vi "Rigol_DG4102.vi"(0 "VISA Refnum in":refnum<visa-resource-name>, 1 "Массив диода":dbl[](array[numeric]), 2 "Масиив детектора":dbl[](array[numeric]), 5 "Количество точек":i32, 7 "Частота (1000 Hz)":dbl=1000.0, 9 "Amplitude (5 Vpp)":dbl=5.0, 12 "Amplitude Unit (0: Vpp)":i32(ring) items=["Vpp", "Vrms", "dBm"], 13 "Amplitude Unit (0: Vpp) 2":i32(ring) items=["Vpp", "Vrms", "dBm"], 14 "Amplitude (5 Vpp) 2":dbl=5.0) -> (3 "VISA resource name out":refnum<visa-resource-name>, 4 "Выход на канал 1":string, 6 "Выход на канал 2":string)   [LabVIEW 2012]
uses:
  RIGOL DG4000 Series.lvlib
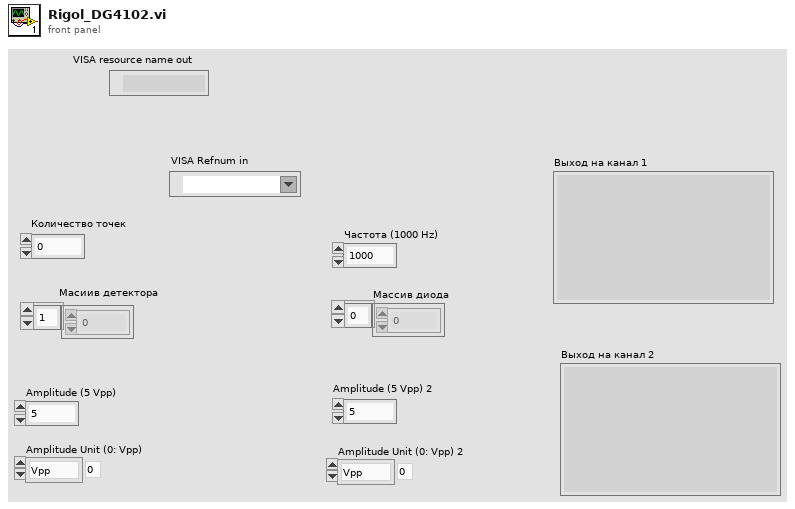
[diagram p1: front panel]
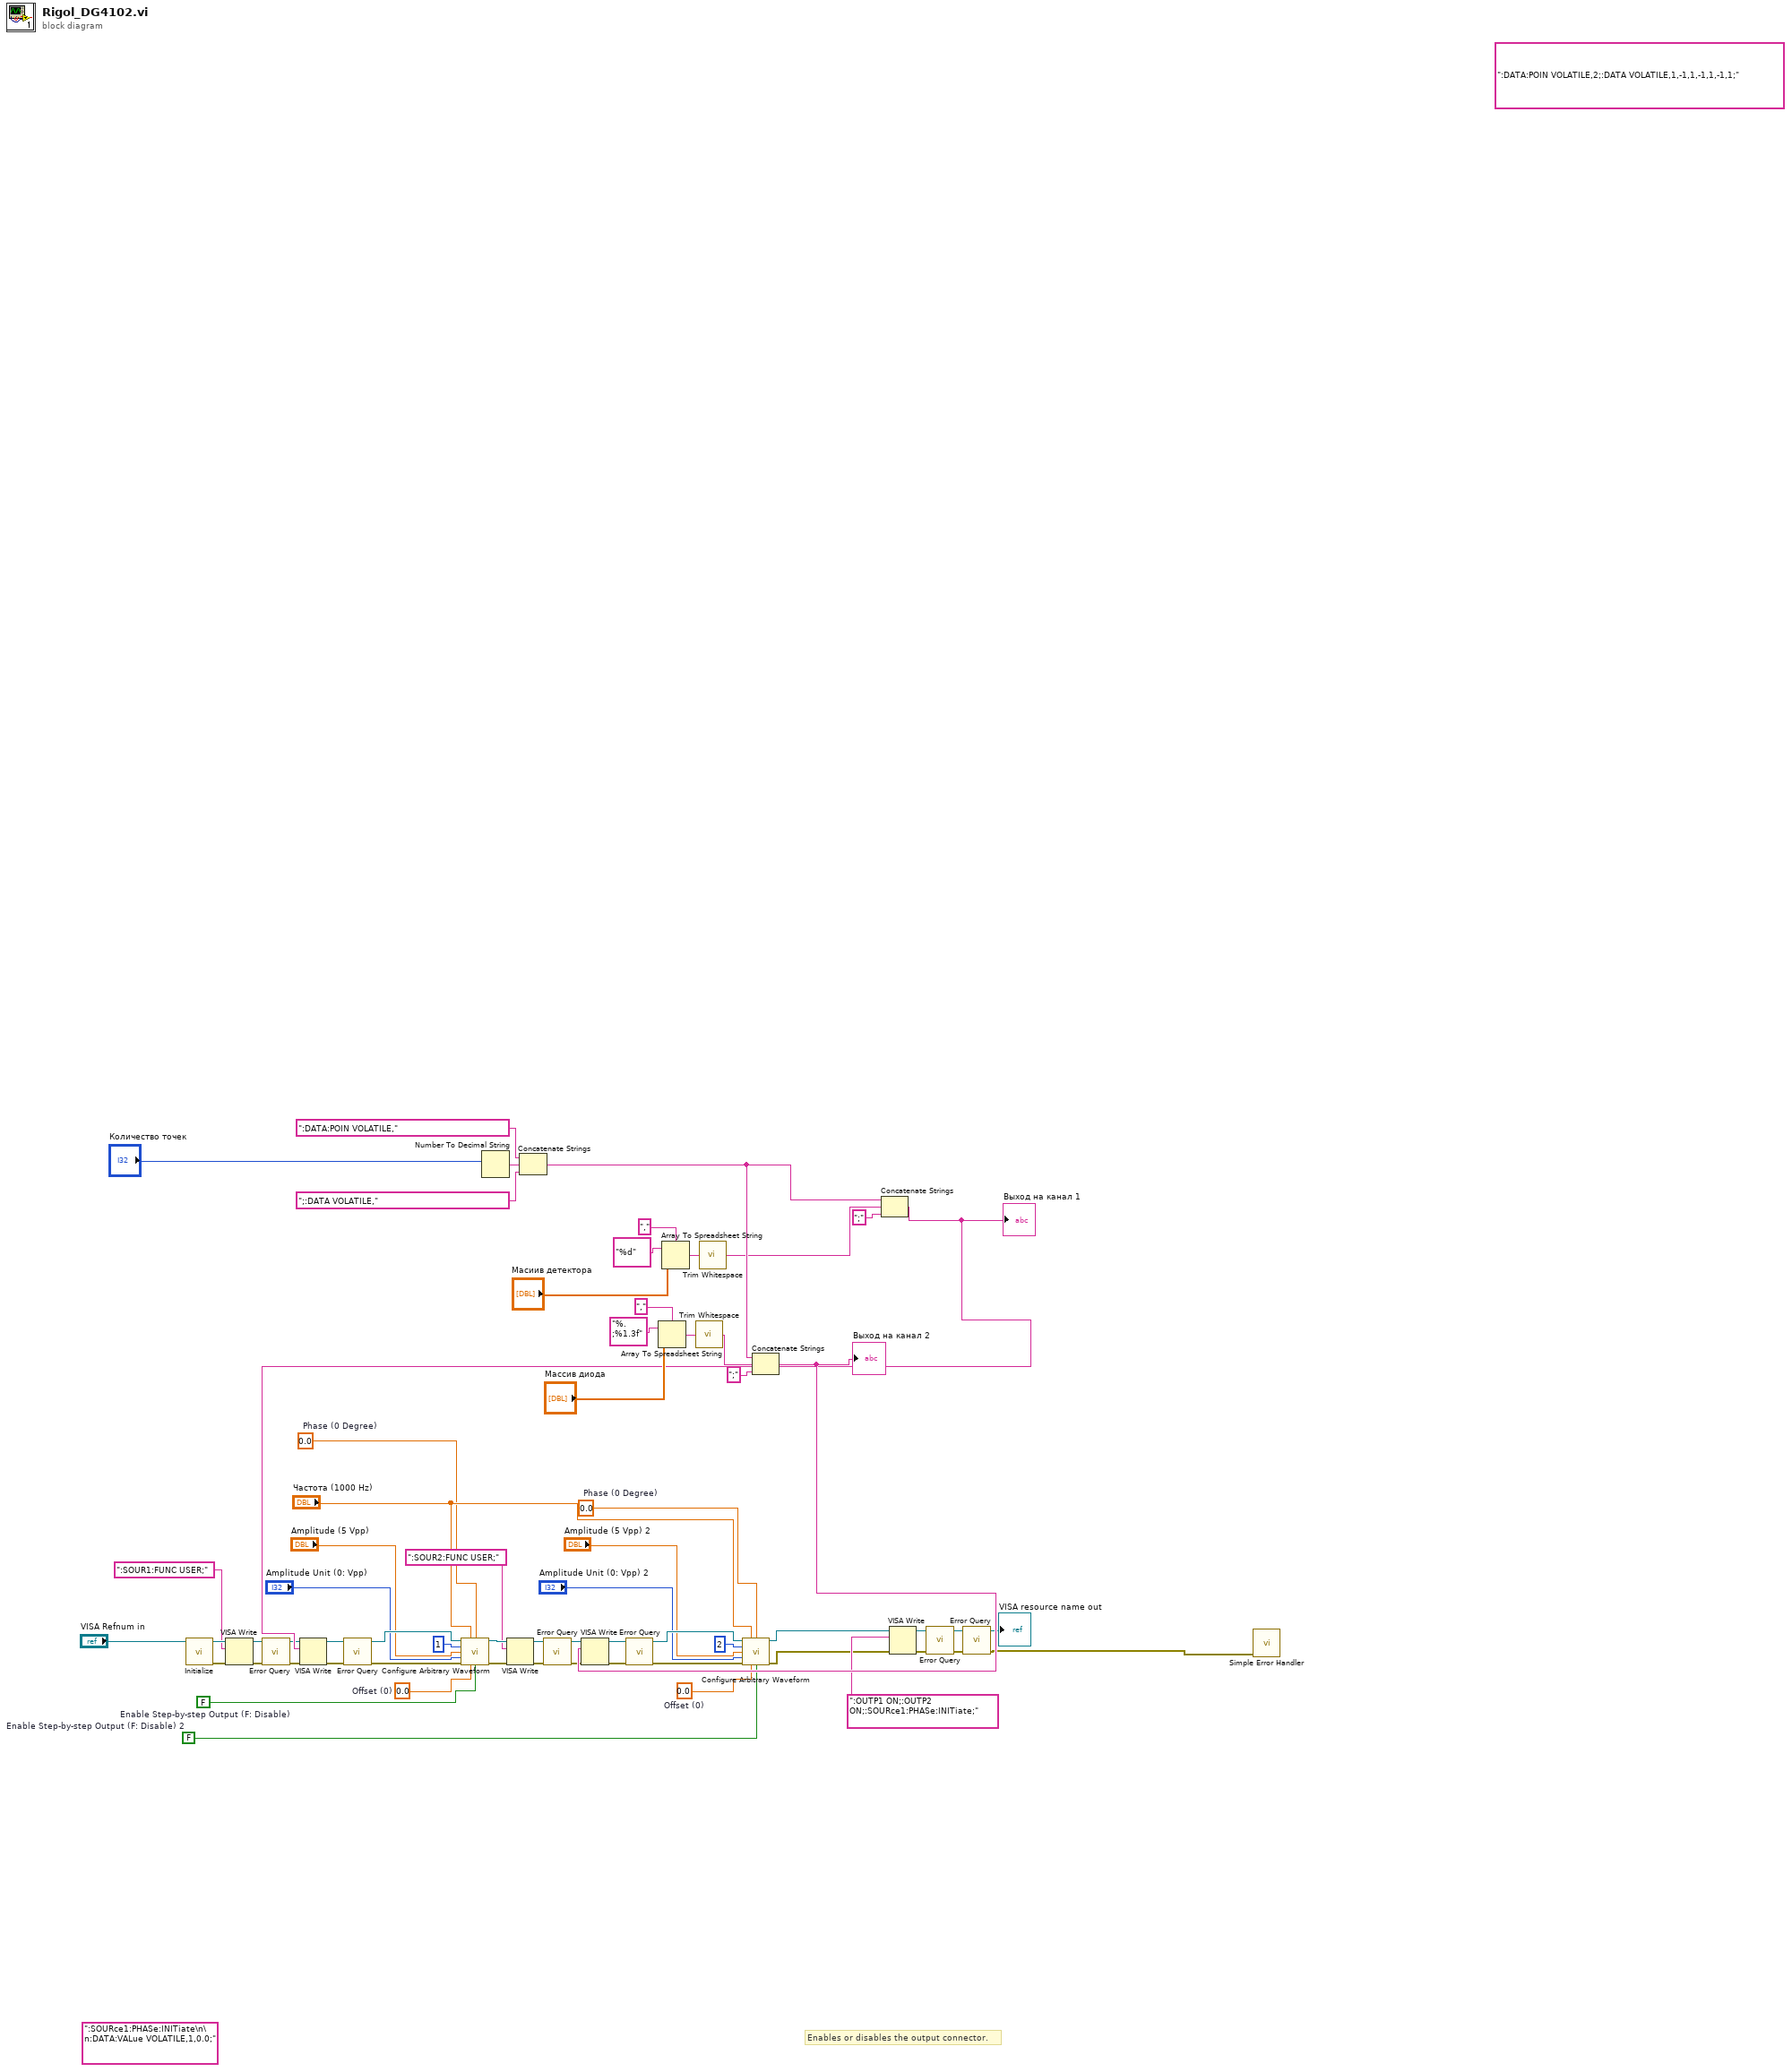
[diagram p0: block diagram]
diagram:
  w44 = FALSE  # Enable Step-by-step Output (F: Disable) 2
  w43 = FALSE  # Enable Step-by-step Output (F: Disable)
  w42 = 0.0  # Offset (0)
  w41 = 0.0  # Phase (0 Degree)
  w40 = 0.0  # Offset (0)
  w39 = 0.0  # Phase (0 Degree)
  (unwired) ":SOURce1:PHASe:INITiate\n\n:DATA:VALue VOLATILE,1,0.0;"
  (unwired) ":DATA:POIN VOLATILE,2;:DATA VOLATILE,1,-1,1,-1,1,-1,1;"
  # "Enables or disables the output connector."
  n1 = call "Initialize.vi"("VISA resource name"="VISA Refnum in") -> ("error out"=w29:errorcluster, "VISA resource name out"=w28:refnum<visa-resource-name>)  [unwired: 4 in, 5 out]
  n2 = VISA Write(VISA resource name=w28, write buffer=":SOUR1:FUNC USER;", error in (no error)=w29) -> (VISA resource name out=w4:refnum<visa-resource-name>, error out=w6:errorcluster)  [unwired: 1 out]
  n3 = call "Error Query.vi"("error in (no error)"=w6, "VISA resource name"=w4) -> ("error out"=w12:errorcluster, "VISA resource name out"=w9:refnum<visa-resource-name>)  [unwired: 8 out]
  n4 = Number To Decimal String(number="Количество точек") -> (decimal integer string=w59:string)  [unwired: 1 in]
  n5 = Concatenate Strings(":DATA:POIN VOLATILE,", w59, ";:DATA VOLATILE,") -> (w63:string)
  n6 = Array To Spreadsheet String(delimiter (Tab)=",", array="Массив диода", 3:"%.;%1.3f") -> (spreadsheet string=w55:string)
  n7 = Array To Spreadsheet String(delimiter (Tab)=",", array="Масиив детектора", 3:"%d") -> (spreadsheet string=w49:string)
  n8 = call <vilib>:"Trim Whitespace.vi"("string"=w55) -> ("trimmed string"=w56:string)  [unwired: 1 in]
  n9 = call <vilib>:"Trim Whitespace.vi"("string"=w49) -> ("trimmed string"=w51:string)  [unwired: 1 in]
  n10 = Concatenate Strings(w63, w56, ";" ("delimiter (Tab)")) -> (w58:string)
  "Выход на канал 2" <- w58
  n11 = Concatenate Strings(w63, w51, ";" ("delimiter (Tab)")) -> (w57:string)
  "Выход на канал 1" <- w57
  n12 = VISA Write(VISA resource name=w9, write buffer=w57, error in (no error)=w12) -> (VISA resource name out=w10:refnum<visa-resource-name>, error out=w13:errorcluster)  [unwired: 1 out]
  n13 = call "Error Query.vi"("error in (no error)"=w13, "VISA resource name"=w10) -> ("error out"=w14:errorcluster, "VISA resource name out"=w11:refnum<visa-resource-name>)  [unwired: 8 out]
  n14 = call "Configure Arbitrary Waveform.vi"("VISA resource name"=w11, "Frequency (1000 Hz)"="Частота (1000 Hz)", "Phase (0 Degree)"=w39, "Output Channel (1: Channel 1)"=1, "Amplitude (5 Vpp)"="Amplitude (5 Vpp)", "Amplitude Unit (0: Vpp)"="Amplitude Unit (0: Vpp)", "error in (no error)"=w14, "Offset (0)"=w40, "Enable Step-by-step Output (F: Disable)"=w43) -> ("VISA resource name out"=w26:refnum<visa-resource-name>, "error out"=w27:errorcluster)  [unwired: 5 in]
  n15 = VISA Write(VISA resource name=w26, write buffer=":SOUR2:FUNC USER;", error in (no error)=w27) -> (VISA resource name out=w15:refnum<visa-resource-name>, error out=w17:errorcluster)  [unwired: 1 out]
  n16 = call "Error Query.vi"("error in (no error)"=w17, "VISA resource name"=w15) -> ("error out"=w23:errorcluster, "VISA resource name out"=w20:refnum<visa-resource-name>)  [unwired: 8 out]
  n17 = VISA Write(VISA resource name=w20, write buffer=w58, error in (no error)=w23) -> (VISA resource name out=w21:refnum<visa-resource-name>, error out=w24:errorcluster)  [unwired: 1 out]
  n18 = call "Error Query.vi"("error in (no error)"=w24, "VISA resource name"=w21) -> ("error out"=w25:errorcluster, "VISA resource name out"=w22:refnum<visa-resource-name>)  [unwired: 8 out]
  n19 = call "Configure Arbitrary Waveform.vi"("VISA resource name"=w22, "Frequency (1000 Hz)"="Частота (1000 Hz)", "Phase (0 Degree)"=w41, "Output Channel (1: Channel 1)"=2, "Amplitude (5 Vpp)"="Amplitude (5 Vpp) 2", "Amplitude Unit (0: Vpp)"="Amplitude Unit (0: Vpp) 2", "error in (no error)"=w25, "Offset (0)"=w42, "Enable Step-by-step Output (F: Disable)"=w44) -> ("VISA resource name out"=w34:refnum<visa-resource-name>, "error out"=w35:errorcluster)  [unwired: 5 in]
  n20 = VISA Write(VISA resource name=w34, write buffer=":OUTP1 ON;:OUTP2 ON;:SOURce1:PHASe:INITiate;", error in (no error)=w35) -> (VISA resource name out=w32:refnum<visa-resource-name>, error out=w33:errorcluster)  [unwired: 1 out]
  n21 = call "Error Query.vi"("error in (no error)"=w33, "VISA resource name"=w32) -> ("error out"=w37:errorcluster, "VISA resource name out"=w38:refnum<visa-resource-name>)  [unwired: 8 out]
  n22 = call "Error Query.vi"("error in (no error)"=w37, "VISA resource name"=w38) -> ("error out"=w2:errorcluster, "VISA resource name out"=→"VISA resource name out":refnum<visa-resource-name>)  [unwired: 8 out]
  n23 = call <vilib>:"Simple Error Handler.vi"("error in (no error)"=w2) -> ()  [unwired: 1 in, 8 out]
